vi "CT_AppendStringError.vi"(1 "Append String":string, 2 "Error In":errorcluster) -> (0 "Error Out":errorcluster)   [LabVIEW 2016]
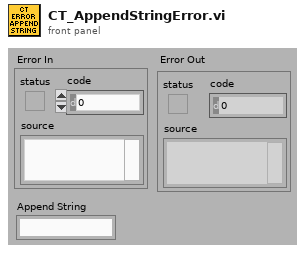
[diagram p1: front panel]
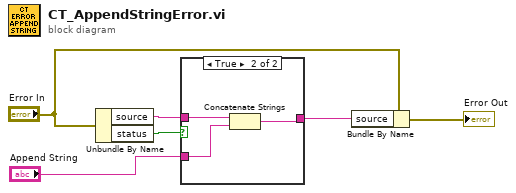
[diagram p0: block diagram]
diagram:
  n1 = Unbundle By Name("Error In") -> ("source"=w4:string, "status"=w2:bool)
  n2 = case shown="True" w2 {
    tunnel: w4 -> [w7 w10]
    tunnel: "Append String" -> [_ w9]
    tunnel: [w7 w8] -> w1
    frame False {
    }
    frame True {
      n3 = Concatenate Strings(w10, w9) -> (w8:string)
    }
  }
  n4 = Bundle By Name(cluster="Error In", "source"=w1) -> (→"Error Out":errorcluster)
